vi "4 channels no handoff (MOSFET).vi"() -> ()   [LabVIEW 2018]
panel:
  out "Blue":bool
  in  "Loop Time (ms)":u32=50
  in  "U":bool
  out "Yellow":bool
  out "Orange":bool
  out "Pink":bool
  in  "stop":bool
  # "TO RIGHT"
  # "TO LEFT"
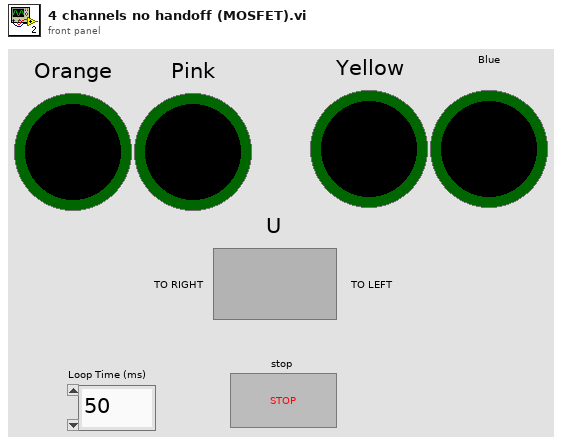
[diagram p1: front panel]
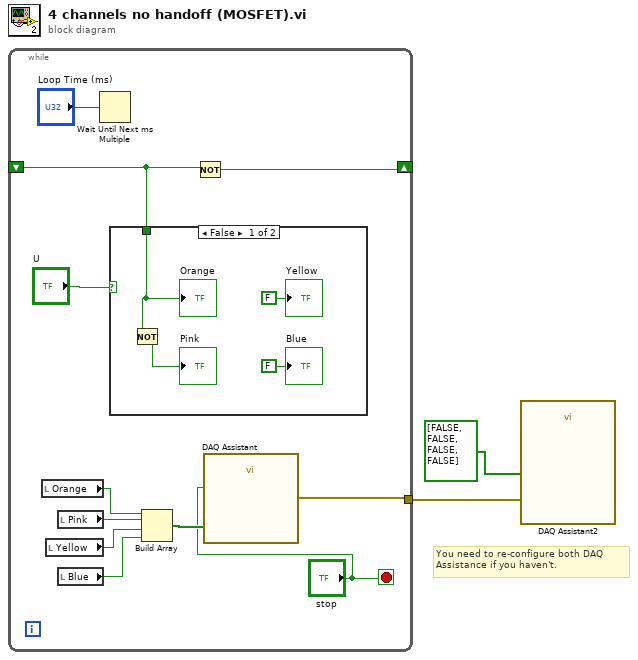
[diagram p0: block diagram]
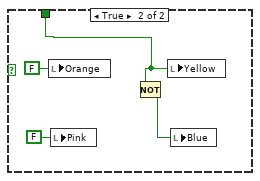
[diagram p2: hidden frame]
diagram:
  # "You need to re-configure both DAQ \nAssistance if you haven't."
  n1 = while {
    shift-right: [w12] -> _
    shift-left: _ -> [w10]
    tunnel: [w3] -> w2
    stop <- "stop" stop-if-true
    n2 = local read "Orange"() -> (w9:bool)
    n3 = local read "Yellow"() -> (w7:bool)
    n4 = local read "Pink"() -> (w8:bool)
    n5 = local read "Blue"() -> (w6:bool)
    n6 = Wait Until Next ms Multiple(millisecond multiple="Loop Time (ms)") -> ()  [unwired: 1 out]
    n7 = case shown="False" "U" {
      tunnel: w10 -> [w15 w21]
      frame False {
        n8 = Not(x=w15) -> (.not. x?=→"Pink":bool)
        "Orange" <- w15
        "Yellow" <- FALSE ("Yellow")
        "Blue" <- FALSE ("Blue")
      }
      frame True {
        n9 = local write "Orange"(FALSE ("Orange")) -> ()
        n10 = local write "Pink"(FALSE ("Pink")) -> ()
        n11 = Not(x=w21) -> (.not. x?=w18:bool)
        n12 = local write "Yellow"(w21) -> ()
        n13 = local write "Blue"(w18) -> ()
      }
    }
    n14 = Build Array(w9, w8, w7, w6) -> (w5:bool[])
    n15 = Not(x=w10) -> (.not. x?=w12:bool)
    n16 = call "DAQ Assistant"("data"=w5, "stop (T)"="stop") -> ("error out"=w3:errorcluster)  [unwired: 16 in, 1 out]
  }
  n17 = call "DAQ Assistant2"("data"=bool[] [FALSE, FALSE, FALSE, FALSE], "error in"=w2) -> ()  [unwired: 16 in, 2 out]
